vi "S2C_PCIe1762H_Proc_DigitalWriteLocal.vi"(8 "Error In":errorcluster, 9 "ExeRef":refnum<vi>, 11 "Q-Ref":refnum<queue>) -> (0 "Error Out":errorcluster, 3 "Command":string)   [LabVIEW 2024]
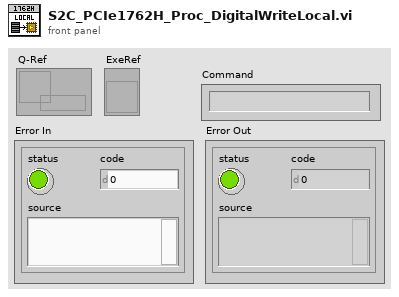
[diagram p1: front panel]
types:
  T1 = cluster{"FootSwitchWr":u16, "WriteState":bool, "P1C3Exe":bool}
  T2 = cluster{"Caller-Q":refnum<queue>, "Command":string, "Return":string, "Data":variant, "Timeout":dbl}
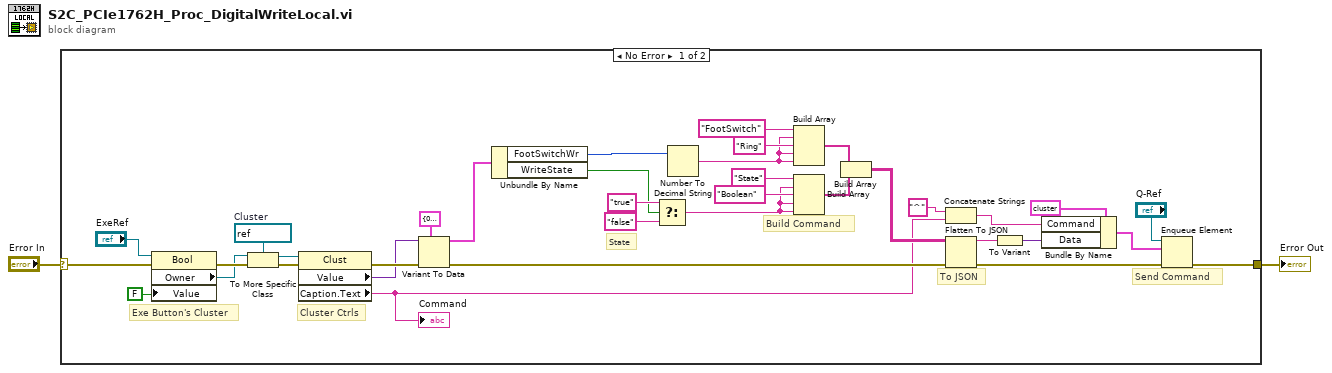
[diagram p0: block diagram]
diagram:
  n1 = case shown="No Error" "Error In" {
    selector: "Error In" -> [w32 w39]
    tunnel: [w31 w39] -> w1
    frame No Error {
      w35 = refnum<vi> refnum  # Cluster
      # "Build Command"
      # "State"
      # "Send Command"
      # "To JSON"
      # "Cluster Ctrls"
      # "Exe Button's Cluster"
      n2 = property class="Bool"(reference="ExeRef", error in=w32, "Value"=FALSE) -> (error out=w37:errorcluster, "Owner"=w36:refnum<vi>)  [unwired: 1 out]
      n3 = To More Specific Class(target class=w35, reference=w36, error in=w37) -> (specific class reference=w33:refnum<vi>, error out=w34:errorcluster)
      n4 = property class="Clust"(reference=w33, error in=w34) -> (error out=w30:errorcluster, "Value"=w29:variant, "Caption.Text"=w8:string)  [unwired: 1 out]
      "Command" <- w8
      n5 = Variant To Data(error in=w30, type=T1 {"FootSwitchWr"=0, "WriteState"=FALSE, "P1C3Exe"=TRUE} ("Write"), Variant=w29) -> (data=w28:T1, error out=w17:errorcluster)
      n6 = Unbundle By Name(w28) -> ("FootSwitchWr"=w7:u16, "WriteState"=w5:bool)
      n7 = Select(t="true", s=w5, f="false") -> (s? t:f=w12:string)
      n8 = Number To Decimal String(number=w7) -> (decimal integer string=w6:string)  [unwired: 1 in]
      n9 = Build Array("FootSwitch" ("element"), w6, "Ring" ("element"), w6, w6) -> (w11:string[])
      n10 = Build Array("State" ("element"), w12, "Boolean" ("element"), w12, w12) -> (w10:string[])
      n11 = Build Array(w11, w10) -> (w9:string[][])
      n12 = Concatenate Strings("^" ("string"), w8) -> (w24:string)
      n13 = Flatten To JSON(anything=w9, error in (no error)=w17) -> (JSON string=w26:string, 11:w27:errorcluster)  [unwired: 1 in]
      n14 = To Variant(anything=w26) -> (Variant=w22:variant)
      n15 = Bundle By Name(cluster=T2 {"Caller-Q"=refnum, "Command"="", "Return"="None", "Data"=variant, "Timeout"=10.0} ("element"), "Command"=w24, "Data"=w22) -> (w21:T2)
      n16 = Enqueue Element(queue="Q-Ref", element=w21, error in (no error)=w27) -> (error out=w31:errorcluster)  [unwired: 1 in, 2 out]
    }
    frame Error {
    }
  }
  "Error Out" <- w1
